vi "Get Windows Process Memory Usage.vi"(8 "Error In":errorcluster) -> (0 "Error Out":errorcluster, 1 "Process Summary":string[][](table), 2 "Labview StartTime":timestamp, 3 "Memory Used By This Process - Labview (KB)":dbl, 4 "Memory Usage Total (KB)":i64, 6 "Number of processes":i32)   [LabVIEW 2014]
panel:
  out "Array String":string[][](array[string])
  out "Process Name":string[](array[string])
  out "Process ID":i32[](array[numeric])
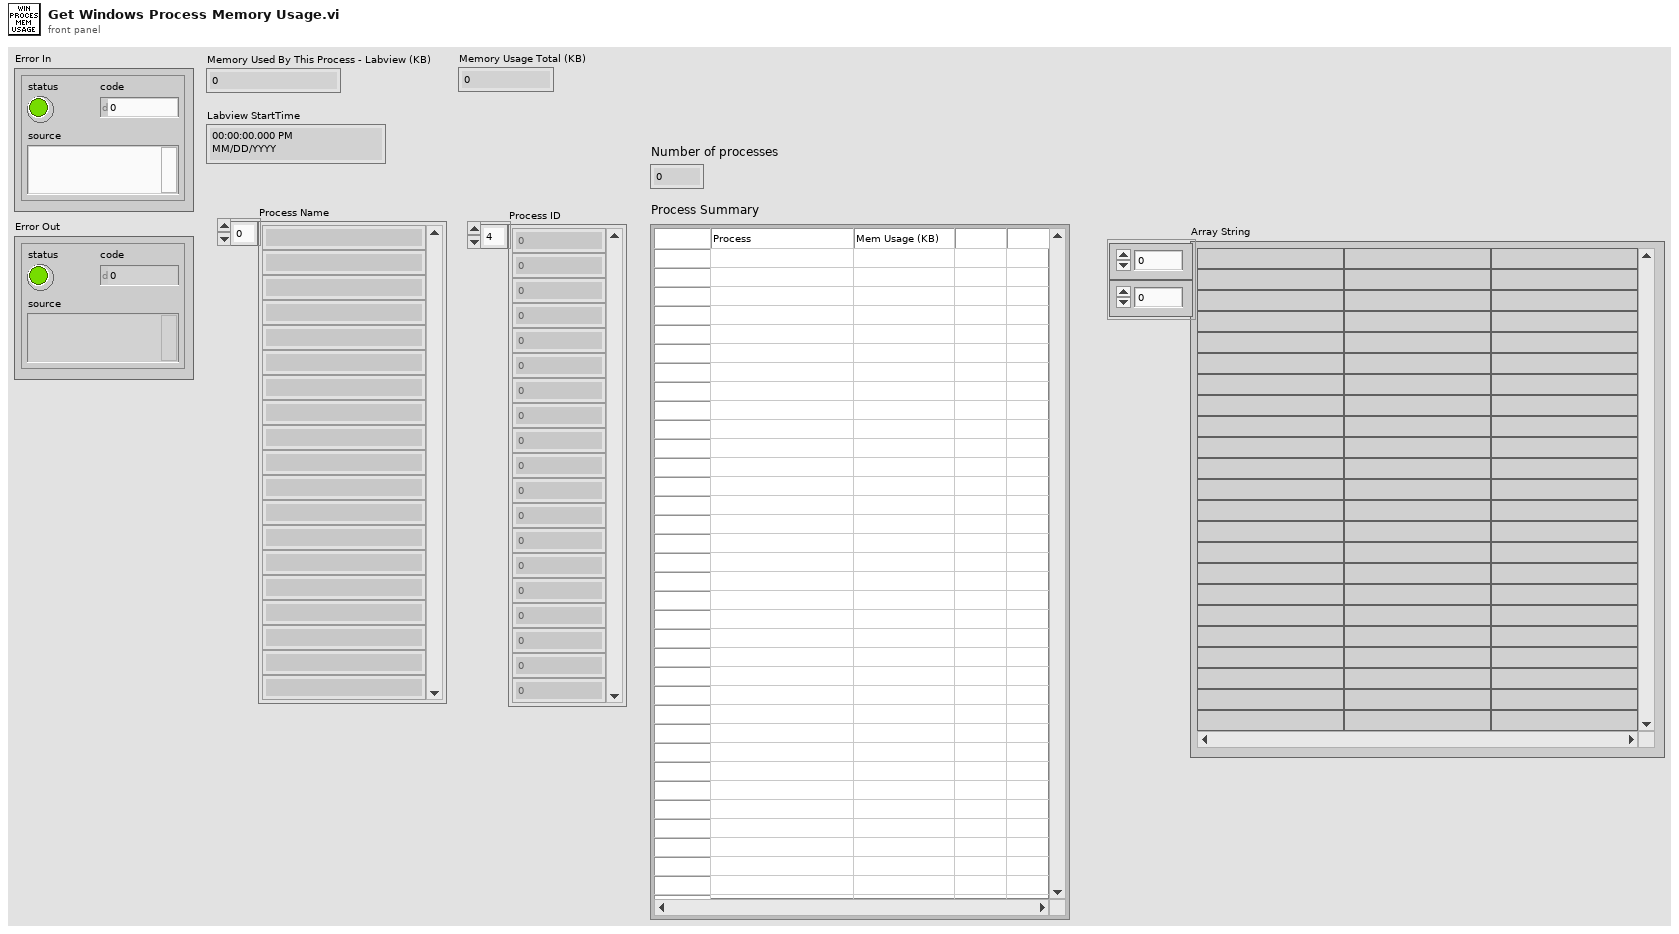
[diagram p1: front panel]
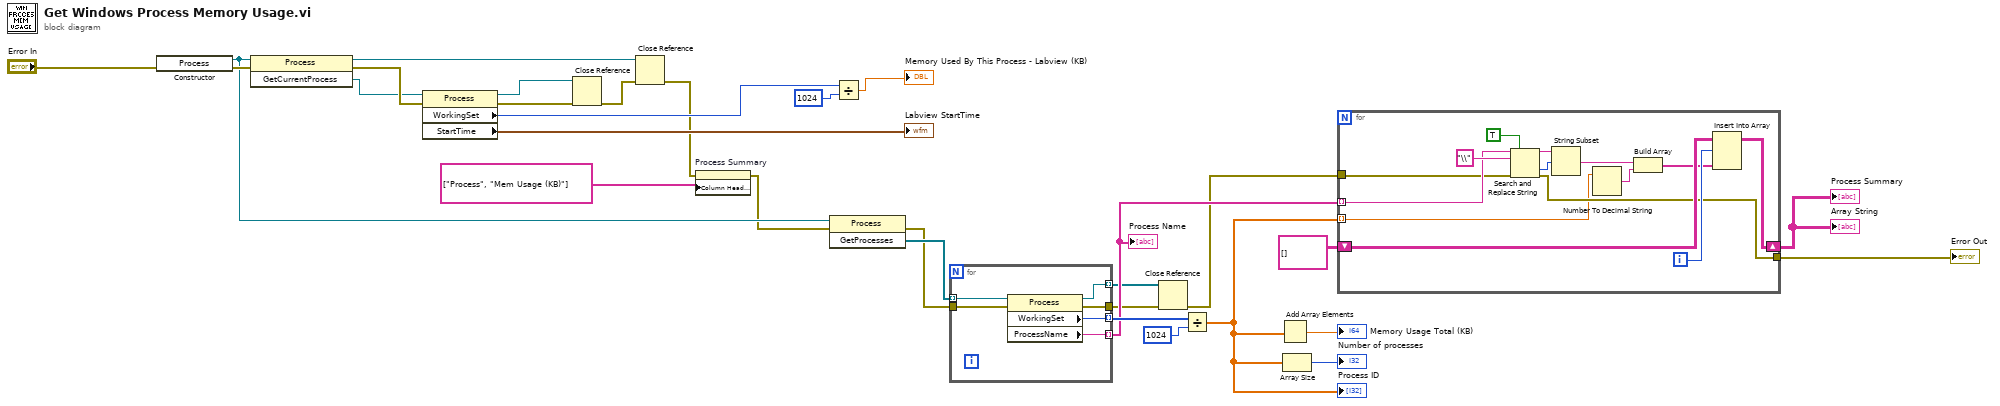
[diagram p0: block diagram]
diagram:
  n1 = constructor class="Process"(error in="Error In") -> (reference out=w11:refnum<k24>, error out=w23:errorcluster)  [unwired: 2 in, 1 out]
  n2 = invoke class="Process" method="GetCurrentProcess"(reference=w11, error in=w23) -> (reference out=w10:refnum<k24>, error out=w30:errorcluster, "GetCurrentProcess"=w9:refnum<k24>)  [unwired: 1 in]
  n3 = property class="Process"(reference=w9, error in=w30) -> (reference out=w27:refnum<k24>, error out=w26:errorcluster, "WorkingSet"=w24:i32, "StartTime"=→"Labview StartTime":timestamp)
  n4 = Close Reference(reference=w27, error in (no error)=w26) -> (error out=w28:errorcluster)
  n5 = Close Reference(reference=w10, error in (no error)=w28) -> (error out=w2:errorcluster)
  n6 = property on="Process Summary" class="Tbl (strict)"(error in=w2, "Column Header Strings[]"=string[] ["Process", "Mem Usage (KB)"] ("new element/subarray")) -> (error out=w3:errorcluster)  [unwired: 1 in, 1 out]
  n7 = invoke class="Process" method="GetProcesses"(reference=w11, error in=w3) -> (error out=w5:errorcluster, "GetProcesses"=w22:refnum<k24>[])  [unwired: 1 in, 1 out]
  n8 = Divide(x=w24, y=i64 1024) -> (x/y=→"Memory Used By This Process - Labview (KB)":dbl)
  n9 = for {
    tunnel: w22 -> [w36] mode=indexing
    tunnel: [w35] -> w20 mode=indexing
    tunnel: [w34] -> w15 mode=indexing
    tunnel: [w33] -> w12 mode=indexing
    tunnel: [w32] -> w6
    tunnel: w5 -> [w31]
    n10 = property class="Process"(reference=w36, error in=w31) -> (reference out=w33:refnum<k24>, error out=w32:errorcluster, "WorkingSet"=w35:i32, "ProcessName"=w34:string)
  }
  "Process Name" <- w15
  n11 = Close Reference(reference=w12, error in (no error)=w6) -> (error out=w4:errorcluster)
  n12 = Divide(x=w20, y=i64 1024) -> (x/y=w14:dbl[])
  "Process ID" <- w14
  n13 = Add Array Elements(numeric array=w14) -> (sum=→"Memory Usage Total (KB)":dbl)
  n14 = Array Size(array=w14) -> (size(s)=→"Number of processes":i32)
  n15 = for {
    tunnel: w15 -> [w46] mode=indexing
    shift-right: [w40] -> w1
    shift-left: string[][] [] ("Process Summary") -> [w42]
    tunnel: w4 -> [w39]
    tunnel: [w38] -> w7
    tunnel: w14 -> [w37] mode=indexing
    i -> [w43]
    n16 = Search and Replace String(replace all?=TRUE ("replace all? (F)"), input string=w46, search string="\\", error in=w39) -> (result string=w44:string, offset past replacement=w47:i32, error out=w38:errorcluster)  [unwired: 4 in, 1 out]
    n17 = String Subset(string=w44, offset (0)=w47) -> (substring=w45:string)  [unwired: 1 in]
    n18 = Number To Decimal String(number=w37) -> (decimal integer string=w50:string)  [unwired: 1 in]
    n19 = Build Array(w45, w50) -> (w41:string[])
    n20 = Insert Into Array(array=w42, index (row)=w43, new element=w41) -> (w40:string[][])  [unwired: 1 in]
  }
  "Process Summary" <- w1
  "Error Out" <- w7
  "Array String" <- w1
